vi "Python_Open.vi"(3 "error in (no error)":errorcluster) -> (10 "error out 2":errorcluster)   [LabVIEW 2021]
doc: "This example demonstrates how to call a Python function and pass integers as arguments. It uses a python function to compute the sum of two integers."
uses:
  Program Files (x86)/National Instruments/LabVIEW 2021/examples/Connectivity/Python/support/PythonVersionsEnum.ctl
  Global_Variables.vi
panel:
  # "e"
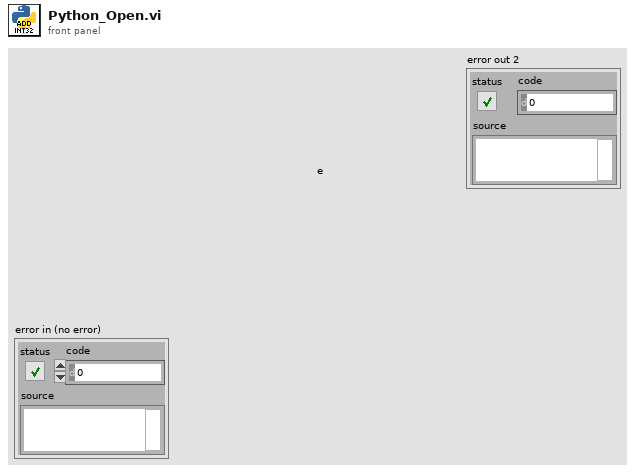
[diagram p1: front panel]
types:
  T1 = typedef "PythonVersionsEnum.ctl" = enum16{"3.6", "3.7", "3.8", "3.9"}
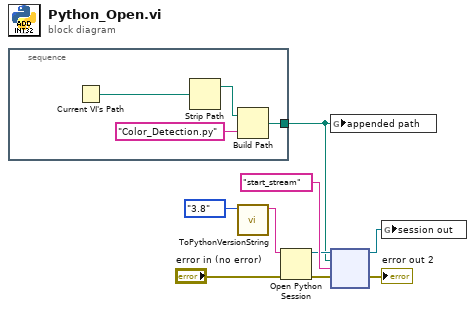
[diagram p0: block diagram]
diagram:
  n1 = stacked-sequence {
    tunnel: [w13] -> w2
    frame #0 {
      n2 = Current VI's Path() -> (path=w10:path)
      n3 = Strip Path(path=w10) -> (stripped path=w11:path)  [unwired: 1 out]
      n4 = Build Path(base path=w11, name or relative path="Color_Detection.py") -> (appended path=w13:path)
    }
  }
  n5 = call "ToPythonVersionString.vi"("python version"=PythonVersionsEnum."3.8") -> ("python version string"=w9:string)  [unwired: 10 in]
  n6 = Open Python Session(python version=w9, 3:"error in (no error)") -> (session out=w6:refnum<k35>, error out=w4:errorcluster)  [unwired: 1 in]
  n7 = global write "Global_Variables.vi" "appended path"(w2) -> ()
  n8 = node(w6, w2, "start_stream" ("function name"), w4) -> (w1:refnum<k35>, →"error out 2":errorcluster)  [unwired: 2 in, 2 out]
  n9 = global write "Global_Variables.vi" "session out"(w1) -> ()
